vi "ScanFromString.vi"() -> ()   [LabVIEW 2021]
panel:
  out "Age":u32
  out "Place":string
  out "Profession":string
  out "Name":string
  in  "String":string="Ankit is an Engineer , Age is 30, Stays in Baroda"
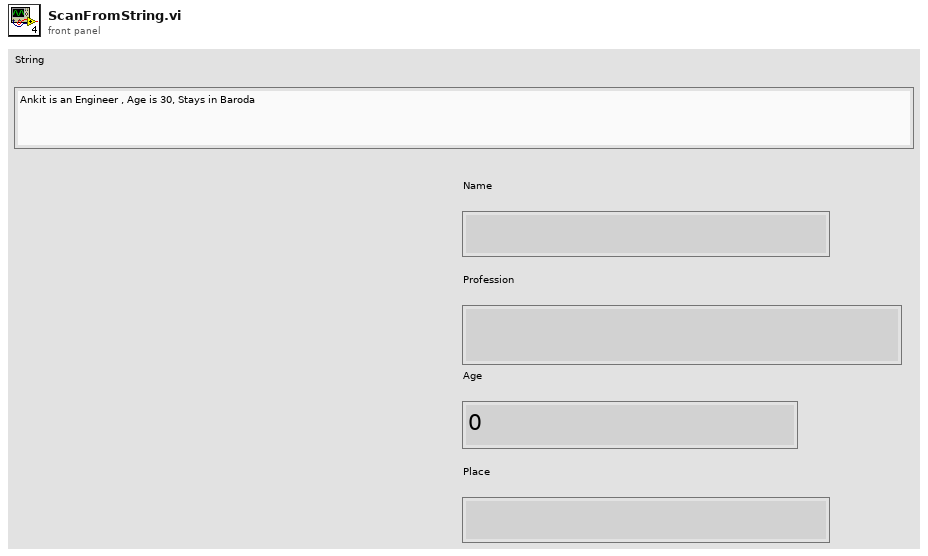
[diagram p1: front panel]
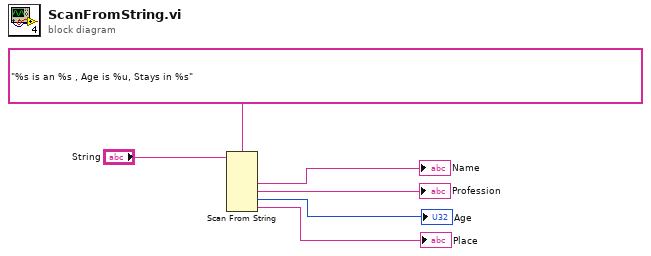
[diagram p0: block diagram]
diagram:
  n1 = Scan From String(format string="%s is an %s , Age is %u, Stays in %s", input string="String") -> (output 1=→"Name":string, output 2=→"Profession":string, output 3=→"Age":u32, output 4=→"Place":string)  [unwired: 6 in, 3 out]
